vi "Custom Constant Dialog.vi"(6 "Project Ref":refnum<vi>, 8 "error in":errorcluster, 9 "App Ref":refnum<vi>, 10 "Theme":bool, 11 "Library in":refnum<vi>) -> (0 "error out":errorcluster, 3 "New Constant VI name":string)   [LabVIEW 2019, in "Panther Dashboard.lvlib"]
uses:
  Panther Dashboard.lvlib
panel:
  out "Current Constant VIs":string[](array[string])
  in  "New Constant VI name (no need to add --constant.vi)":string
  in  "Continue":bool
  in  "Cancel":bool
  # "Constant VIs\n\nIn LabVIEW, constant VIs (virtual instruments) offer a powerful approach to managing fixed values within your application. They function similarly to regular constants on the block diagram, but with a key advantage: centralized editing.\n\nBenefits of Constant VIs:\n\nSingle Point of Editing: Whenever you need to modify the constant value, you only need to edit it in this single VI. Changes will propagate to all instances where the constant VI is used throughout your application. This saves time and ensures consistency.\nImproved Maintainability: By having a dedicated VI for the constant, your code becomes more modular and easier to understand. Other developers can readily identify where specific values are defined.\nError Reduction: The risk of typos or inconsistencies in the constant value across different parts of your application is minimized."
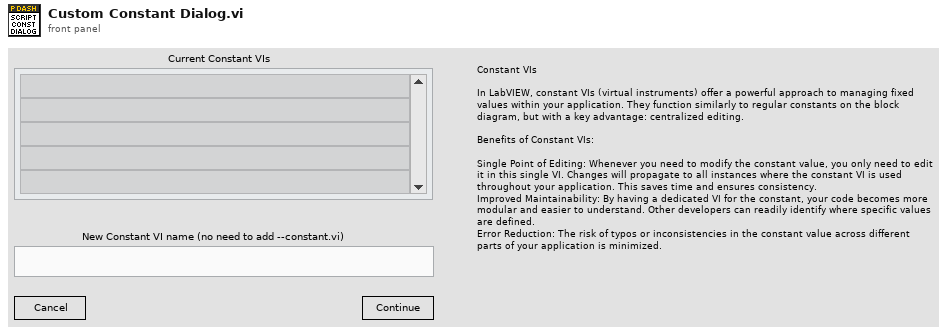
[diagram p1: front panel]
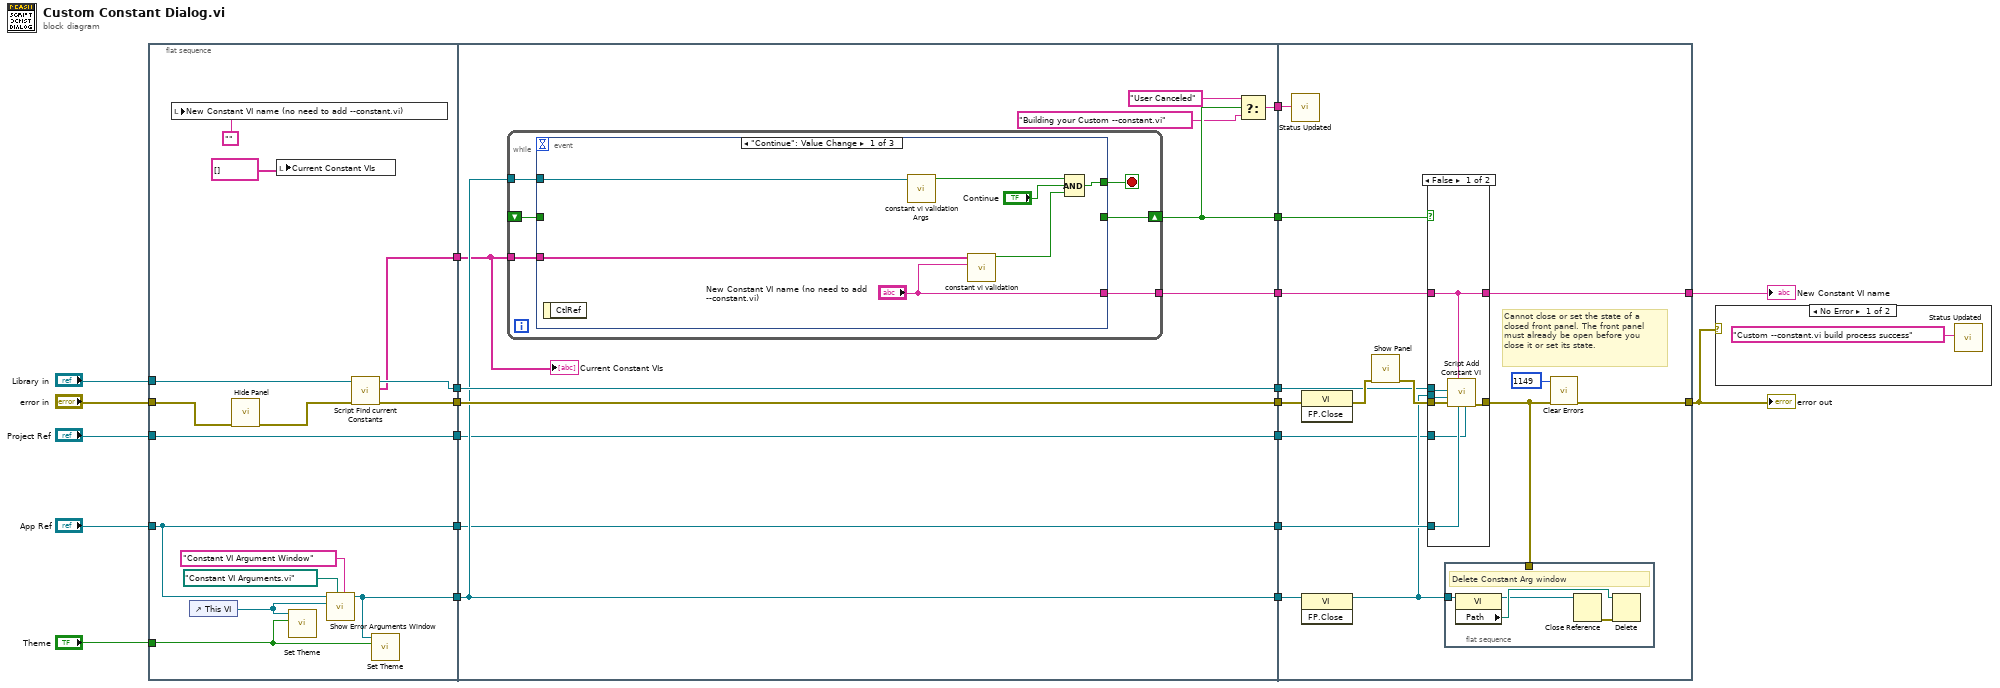
[diagram p0: block diagram]
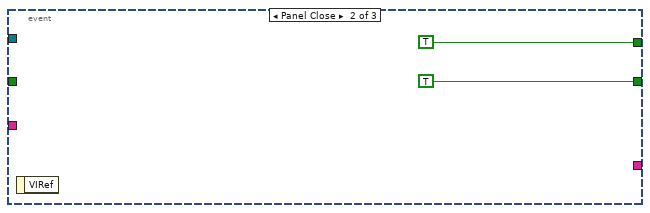
[diagram p3: hidden frame]
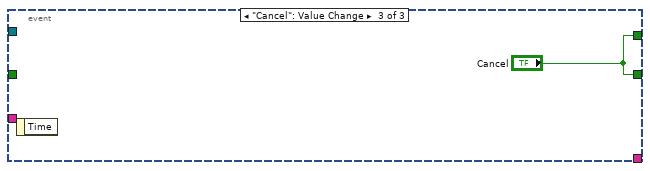
[diagram p4: hidden frame]
diagram:
  n1 = flat-sequence {
    tunnel: "Library in" -> [w33]
    tunnel: "error in" -> [w36]
    tunnel: [w35] -> w20
    tunnel: [w32] -> w14
    tunnel: [w24] -> w13
    tunnel: [w30] -> w11
    tunnel: "App Ref" -> [w26]
    tunnel: "Theme" -> [w29]
    tunnel: [w26] -> w8
    tunnel: [w22] -> w4
    tunnel: "Project Ref" -> [w22]
    tunnel: w20 -> [w47]
    tunnel: [w47] -> w19
    tunnel: [w41] -> w16
    tunnel: [w46] -> w15
    tunnel: w14 -> [w46]
    tunnel: w13 -> [w42]
    tunnel: [w45] -> w12
    tunnel: w11 -> [w45]
    tunnel: w8 -> [w44]
    tunnel: [w44] -> w7
    tunnel: [w43] -> w6
    tunnel: [w39] -> w5
    tunnel: w4 -> [w37]
    tunnel: [w37] -> w2
    tunnel: [w78] -> w18
    tunnel: w19 -> [w77]
    tunnel: w16 -> [w73]
    tunnel: w15 -> [w72]
    tunnel: w12 -> [w71]
    tunnel: w7 -> [w70]
    tunnel: w6 -> [w69]
    tunnel: w5 -> [w67]
    tunnel: w2 -> [w65]
    tunnel: [w64] -> w1
    frame #0 {
      n2 = local write "New Constant VI name (no need to add --constant.vi)"("") -> ()
      n3 = control-ref of="This VI"() -> (w31:refnum<vi>)
      n4 = call "Hide Panel.vi"("error in (no error)"=w36) -> ("error out"=w34:errorcluster)  [unwired: 10 in]
      n5 = local write "Current Constant VIs"(string[] [] ("Current Constant VIs")) -> ()
      n6 = call "Set Theme.vi"("Dark?"=w29, "VI in"=w31) -> ()  [unwired: 10 in]
      n7 = call "Show Error Arguments Window.vi"("Title"="Constant VI Argument Window", "Path"=path "Constant VI Arguments.vi", "Calling VI Ref"=w31, "App Instance"=w26) -> ("Error Arguments Window Ref"=w30:refnum<vi>)  [unwired: 6 in, 1 out]
      n8 = call "Script Find current Constants.vi"("error in"=w34, "Library in"=w33) -> ("error out"=w35:errorcluster, "Constant VIs"=w24:string[], "Library out"=w32:refnum<vi>)  [unwired: 7 in]
      n9 = call "Set Theme.vi"("Dark?"=w29, "VI in"=w30) -> ()  [unwired: 10 in]
    }
    frame #1 {
      n10 = while {
        tunnel: w42 -> [w51]
        tunnel: w45 -> [w50]
        shift-right: [w52] -> w41
        shift-left: _ -> [w49]
        tunnel: [w48] -> w43
        stop <- w53 stop-if-true
        n11 = event shown="[0] \"Continue\": Value Change" {
          selector: _ -> [_ _ _]
          dyn-events: _ -> [_ _ _]
          timeout: _ -> [_ _ _]
          tunnel: [w60 TRUE ("Cancel") "Cancel"] -> w53
          tunnel: [_ TRUE ("Cancel") "Cancel"] -> w52
          tunnel: w51 -> [w57 _ _]
          tunnel: w50 -> [w54 _ _]
          tunnel: w49 -> [_ _ _]
          tunnel: ["New Constant VI name (no need to add --constant.vi)" _ _] -> w48
          event "Continue": Value Change {
            n12 = event-data() -> ()  [unwired: 1 in, 1 out]
            n13 = call "constant vi validation Args.vi"("Constant Argument Window"=w54) -> ("Proceed with Scripting"=w58:bool)  [unwired: 10 in]
            n14 = call "constant vi validation.vi"("New Constant vi name"="New Constant VI name (no need to add --constant.vi)", "Constant VI List"=w57) -> ("Proceed with Scripting"=w56:bool)  [unwired: 9 in]
            n15 = Compound Arithmetic op=AND(w58, "Continue", w56) -> (w60:bool)
          }
          event Panel Close {
            n16 = event-data() -> ()  [unwired: 1 in, 1 out]
          }
          event "Cancel": Value Change {
            n17 = event-data() -> ()  [unwired: 1 in, 1 out]
          }
        }
      }
      n18 = Select(t="User Canceled", s=w41, f="Building your Custom --constant.vi") -> (s? t:f=w39:string)
      "Current Constant VIs" <- w42
    }
    frame #2 {
      # "Cannot close or set the state of a closed front panel. The front panel must already be open before you close it or set its state."
      n19 = call "Status Updated.vi"("Status"=w67) -> ()  [unwired: 10 in, 1 out]
      n20 = invoke class="VI" method="FP.Close"(error in=w77) -> (error out=w75:errorcluster)  [unwired: 2 in, 2 out]
      n21 = invoke class="VI" method="FP.Close"(reference=w71) -> (reference out=w66:refnum<vi>)  [unwired: 2 in, 2 out]
      n22 = call "Show Panel.vi"("error in (no error)"=w75) -> ("error out"=w76:errorcluster)  [unwired: 10 in]
      n23 = case shown="False" w73 {
        tunnel: [w88 w91] -> w74
        tunnel: w76 -> [w89 w91]
        tunnel: w72 -> [w86 _]
        tunnel: w66 -> [w87 _]
        tunnel: w70 -> [w85 _]
        tunnel: w69 -> [w83 w90]
        tunnel: w65 -> [w84 _]
        tunnel: [w83 w90] -> w64
        frame False {
          n24 = call "Script Add Constant VI.vi"("Project Ref"=w84, "App Ref"=w85, "Constant VI Name"=w83, "error in"=w89, "Constant VI Args"=w87, "DQMH Lib Ref"=w86) -> ("error out"=w88:errorcluster)  [unwired: 5 in]
        }
        frame True {
        }
      }
      n25 = flat-sequence {
        tunnel: w66 -> [w81]
        tunnel: w74 -> [_]
        frame #0 {
          # "Delete Constant Arg window"
          n26 = property class="VI"(reference=w81) -> (reference out=w79:refnum<vi>, "Path"=w80:path)  [unwired: 1 in, 1 out]
          n27 = Close Reference(reference=w79) -> (error out=w82:errorcluster)  [unwired: 1 in]
          n28 = Delete(path (use dialog)=w80, error in=w82) -> ()  [unwired: 3 in, 3 out]
        }
      }
      n29 = call <vilib>:"Clear Errors.vi"("error in (no error)"=w74, "specific error code to clear (0: all)"=1149) -> ("error out"=w78:errorcluster)  [unwired: 4 in, 1 out]
    }
  }
  n30 = case shown="No Error" w18 {
    frame No Error {
      n31 = call "Status Updated.vi"("Status"="Custom --constant.vi build process success") -> ()  [unwired: 10 in, 1 out]
    }
    frame Error {
    }
  }
  "error out" <- w18
  "New Constant VI name" <- w1
